vi "Distortion_NI_IMAQdx.vi"() -> ()   [LabVIEW 2017]
uses:
  <vilib>/vision/Calibration.llb/Distortion Model.ctl
  <vilib>/vision/Calibration.llb/Distortion Model Types.ctl
  <vilib>/vision/NI_Vision_Development_Module.lvlib
panel:
  in  "Grid Descriptor":cluster{"X Step":sgl, "Y Step":sgl, "Unit":T1}={"X Step"=5.0, "Y Step"=5.0, "Unit"=enum."Millimeter"}
  out "Original Image":T2(plugin-control)
  out "Corrected Image":T2(plugin-control)
  in  "File Path":path
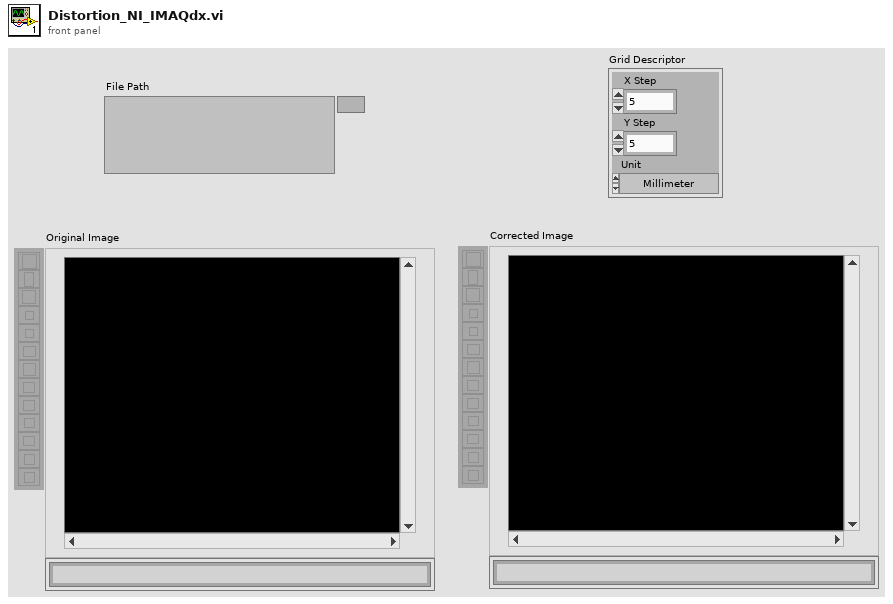
[diagram p1: front panel]
types:
  T1 = typedef "Image Unit" = enum32{"Undefined", "Angström", "Micrometer", "Millimeter", "Centimeter", "Meter", "Kilometer", "Microinch", "Inch", "Feet", "Nautical miles", "Standard miles", "Steps"}
  T2 = typedef "IMAQ Image.ctl" = refnum<image>
  T3 = typedef "Distortion Model.ctl" = cluster{"Distortion Model":T4, "Polynomial Model Setup":cluster{"Radial Coefficient":u32, "Tangential Coefficients ":bool}}
  T4 = typedef "Distortion Model Types.ctl" = i32
  T5 = typedef "Particle Parameters" = i32
  T6 = cluster{"Measurement Parameter":T5, "Range Lower Value":dbl, "Range Upper Value":dbl, "Range":bool, "Measurement Type":bool}[]
  T7 = typedef "Calibration Reference Points.ctl" = cluster{"Pixel Coordinates":cluster{"X":dbl, "Y":dbl}[], "Real World Coordinates":cluster{"X":dbl, "Y":dbl}[], "Unit":T1, "Image Size":cluster{"X":u32, "Y":u32}}
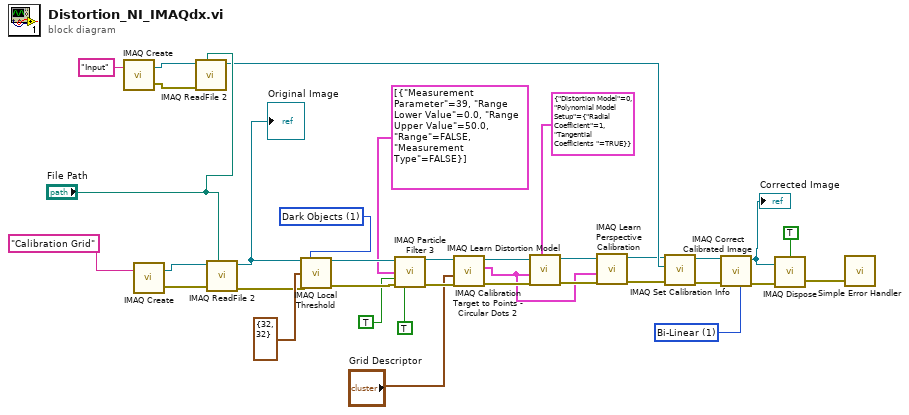
[diagram p0: block diagram]
diagram:
  w6 = u32 1 items=["Zero Order", "Bi-Linear", "Quadratic", "Cubic Spline"] ("Interpolation Type")
  w27 = u32 1 items=["Bright Objects", "Dark Objects"] ("Look For (Bright Objects)")
  n1 = call "IMAQ Create"("Image Name"="Input") -> ("New Image"=w33:T2, "error out"=w34:errorcluster)  [unwired: 4 in]
  n2 = call "IMAQ Create"("Image Name"="Calibration Grid") -> ("New Image"=w29:T2, "error out"=w28:errorcluster)  [unwired: 4 in]
  n3 = call "IMAQ ReadFile 2"("File Path"="File Path", "error in (no error)"=w34, "Image"=w33) -> ("Image Out"=w31:T2)  [unwired: 4 in, 4 out]
  n4 = call "IMAQ ReadFile 2"("File Path"="File Path", "error in (no error)"=w28, "Image"=w29) -> ("error out"=w25:errorcluster, "Image Out"=w2:T2)  [unwired: 4 in, 3 out]
  "Original Image" <- w2
  n5 = call "IMAQ Local Threshold"("Image Src"=w2, "Look For (Bright Objects)"=w27, "Window Size (32x32)"=cluster{"SizeX":i32, "SizeY":i32} {"SizeX"=32, "SizeY"=32}, "error in (no error)"=w25) -> ("Image Dst Out"=w20:T2, "error out"=w24:errorcluster)  [unwired: 10 in]
  n6 = call "IMAQ Particle Filter 3"("Image Src"=w20, "Selection Values"=T6 [{"Measurement Parameter"=39, "Range Lower Value"=0.0, "Range Upper Value"=50.0, "Range"=FALSE, "Measurement Type"=FALSE}], "Keep/Remove Particles (F)"=TRUE, "error in (no error)"=w24, "Reject Border? (F)"=TRUE) -> ("Image Dst Out"=w16:T2, "error out"=w23:errorcluster)  [unwired: 8 in, 1 out]
  n7 = call "IMAQ Calibration Target to Points - Circular Dots 2"("error in (no error)"=w23, "Grid Descriptor"="Grid Descriptor", "Target Image"=w16) -> ("error out"=w22:errorcluster, "Reference Points"=w14:T7, "Target Image (dup)"=w15:T2)  [unwired: 6 in]
  n8 = call "IMAQ Learn Distortion Model"("Distortion Model Setup"=T3 {"Distortion Model"=0, "Polynomial Model Setup"={"Radial Coefficient"=1, "Tangential Coefficients "=TRUE}}, "error in (no error)"=w22, "Reference Points"=w14, "Calibration Template Image"=w15) -> ("error out"=w21:errorcluster, "Calibration Template Image Out"=w13:T2)  [unwired: 6 in]
  n9 = call "IMAQ Learn Perspective Calibration"("error in (no error)"=w21, "Reference Points"=w14, "Calibration Template Image"=w13) -> ("error out"=w10:errorcluster, "Calibration Template Image Out"=w12:T2)  [unwired: 7 in]
  n10 = call "IMAQ Set Calibration Info"("error in (no error)"=w10, "Image Dst"=w31, "Image Src"=w12) -> ("error out"=w7:errorcluster, "Calibrated Image"=w9:T2)  [unwired: 7 in]
  n11 = call "IMAQ Correct Calibrated Image"("Interpolation Type"=w6, "error in (no error)"=w7, "Image Src"=w9) -> ("error out"=w4:errorcluster, "Corrected Image"=w8:T2)  [unwired: 7 in]
  "Corrected Image" <- w8
  n12 = call "IMAQ Dispose"("All Images? (No)"=TRUE, "Image"=w8, "error in (no error)"=w4) -> ("error out"=w3:errorcluster)  [unwired: 3 in]
  n13 = call <vilib>:"Simple Error Handler.vi"("error in (no error)"=w3) -> ()  [unwired: 4 in, 5 out]
